vi "Initialize-object.vi"(8 "error in (no error)":errorcluster, 9 "Panes settings":T1[](array[typedef]), 10 "VI Reference":refnum<vi>) -> (0 "error out":errorcluster, 3 "Panes out":T5)   [LabVIEW 2013, in "HardwareCharacterization.lvlib" / "HC-UI.lvclass"]
uses:
  HC-UI.lvclass
  Panes-reference.ctl
  Pane-settings.ctl
  Pane-names.ctl
  Splitter-settings.ctl
  Splitter-names.ctl
  HC-UI.lvclass/HC-UI.ctl
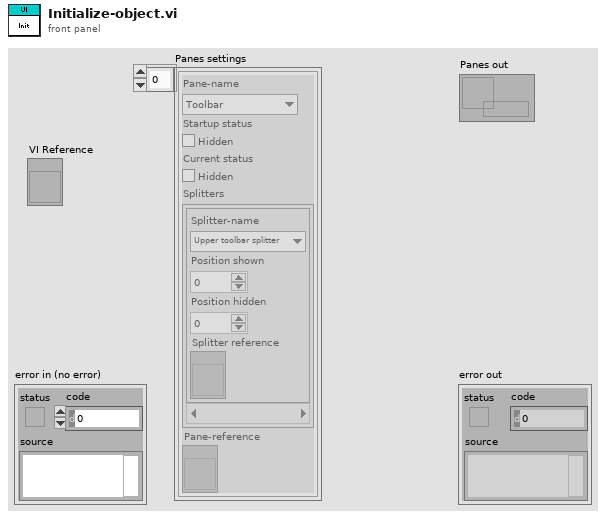
[diagram p1: front panel]
types:
  T1 = typedef "HardwareCharacterization.lvlib/HC-UI.lvclass/Pane-settings.ctl" = cluster{"Pane-name":T2, "Startup status":bool, "Current status":bool, "Splitters":T3[], "Pane-reference":refnum<vi>}
  T2 = typedef "HardwareCharacterization.lvlib/HC-UI.lvclass/Pane-names.ctl" = enum16{"Toolbar", "Help bar", "Toolbar lower border", "Center panel", "Main panel", "Settings panel", "Status bar upper border", "General state bar", "Information bar"}
  T3 = typedef "HardwareCharacterization.lvlib/HC-UI.lvclass/Splitter-settings.ctl" = cluster{"Splitter-name":T4, "Position shown":i32, "Position hidden":i32, "Splitter reference":refnum<vi>}
  T4 = typedef "HardwareCharacterization.lvlib/HC-UI.lvclass/Splitter-names.ctl" = enum16{"Upper toolbar splitter", "Help bar splitter", "Lower toolbar splitter", "Upper status bar splitter", "Lower status bar splitter", "Left status bar splitter", "Settings splitter"}
  T5 = typedef "HardwareCharacterization.lvlib/HC-UI.lvclass/Panes-reference.ctl" = refnum<data-value>
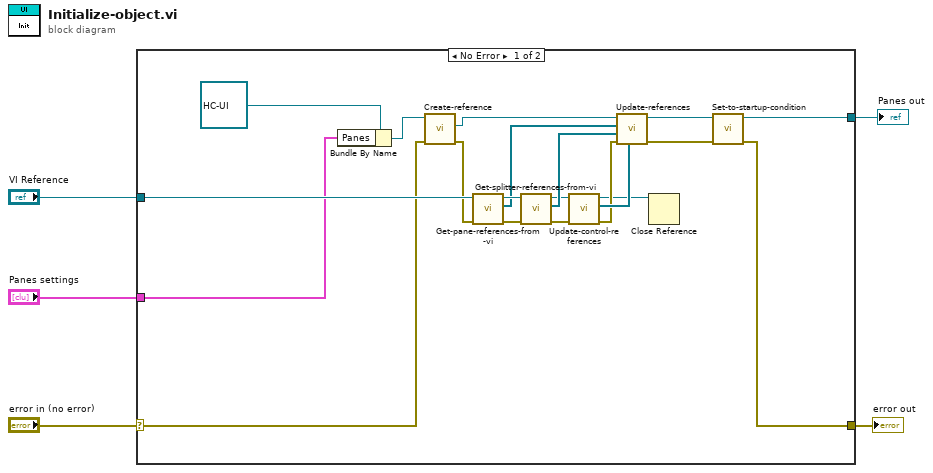
[diagram p0: block diagram]
diagram:
  n1 = case shown="No Error" "error in (no error)" {
    selector: "error in (no error)" -> [w14 w26]
    tunnel: [w13 w26] -> w4
    tunnel: [w12 _] -> w3
    tunnel: "VI Reference" -> [w24 _]
    tunnel: "Panes settings" -> [w11 _]
    frame No Error {
      n2 = Bundle By Name(cluster=refnum<class "HC-UI.lvclass"> refnum ("Panes.lvclass"), "Panes"=w11) -> (w22:refnum<class "HC-UI.lvclass">)
      n3 = call "Create-reference.vi"("error in (no error)"=w14, "Panes in"=w22) -> ("error out"=w21:errorcluster, "Panes reference"=w17:T5)  [unwired: 7 in, 1 out]
      n4 = call "Get-pane-references-from-vi.vi"("error in (no error)"=w21, "VI Reference"=w24) -> ("error out"=w20:errorcluster, "Sorted pane references"=w19:refnum<vi>[], "VI Reference out"=w23:refnum<vi>)  [unwired: 7 in]
      n5 = call "Get-splitter-references-from-vi.vi"("error in (no error)"=w20, "VI Reference"=w23) -> ("error out"=w9:errorcluster, "Sorted splitter references"=w18:refnum<vi>[], "VI Reference out"=w10:refnum<vi>)  [unwired: 7 in]
      n6 = call "Update-control-references.vi"("error in (no error)"=w9, "VI Reference"=w10) -> ("error out"=w7:errorcluster, "Control refs"=w8:refnum<vi>[], "VI Reference"=w6:refnum<vi>)  [unwired: 7 in]
      n7 = call "Update-references.vi"("Control refs"=w8, "error in (no error)"=w7, "Sorted splitter references"=w18, "Sorted pane references"=w19, "Panes in"=w17) -> ("error out"=w15:errorcluster, "Panes out"=w16:T5)  [unwired: 5 in]
      n8 = Close Reference(reference=w6) -> ()  [unwired: 1 in, 1 out]
      n9 = call "Set-to-startup-condition.vi"("error in (no error)"=w15, "Panes in"=w16) -> ("error out"=w13:errorcluster, "Panes out"=w12:T5)  [unwired: 8 in]
    }
    frame Error {
    }
  }
  "error out" <- w4
  "Panes out" <- w3
